vi "Fetch Measurement (Spectrum Emission Mask).vi"(0 "VISA resource name":refnum<visa-resource-name>, 5 "Timeout (10000 ms)":u32=10000, 11 "error in (no error)":errorcluster) -> (4 "VISA resource name out":refnum<visa-resource-name>, 6 "Measurement Data":dbl[](array[numeric]), 15 "error out":errorcluster)   [LabVIEW 2022 SP3, in "Agilent N934X Series.lvlib"]
doc: "Returns the results of last measurement (Spectrum Emission Mask) and does not initiate data acquisition.\n\nNote:\n\nUse this VI only with other low-level VIs. The high-level VIs automatically incorporate this functionality. This VI does not check the instrument status.\n\nThis VI is only applicable for N9321C, N9322C, N9323C, N9324C models."
uses:
  <instrlib>/Agilent N934X Series/Agilent N934X Series.lvlib
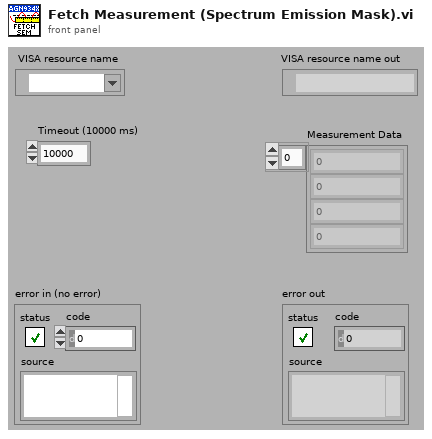
[diagram p1: front panel]
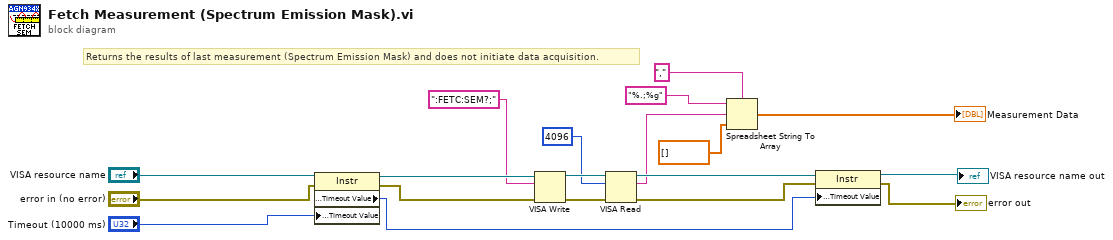
[diagram p0: block diagram]
diagram:
  # "Returns the results of last measurement (Spectrum Emission Mask) and does not initiate data acquisition."
  n1 = property on="Property Node" class="Instr"(reference="VISA resource name", error in="error in (no error)", "General Settings:Timeout Value"="Timeout (10000 ms)") -> (reference out=w17:refnum<visa-resource-name>, error out=w16:errorcluster, "General Settings:Timeout Value"=w18:u32)
  n2 = VISA Write(VISA resource name=w17, write buffer=":FETC:SEM?;", error in (no error)=w16) -> (VISA resource name out=w7:refnum<visa-resource-name>, error out=w8:errorcluster)  [unwired: 1 out]
  n3 = VISA Read(VISA resource name=w7, byte count=u32 4096, error in (no error)=w8) -> (VISA resource name out=w15:refnum<visa-resource-name>, read buffer=w5:string, error out=w12:errorcluster)  [unwired: 1 out]
  n4 = Spreadsheet String To Array(delimiter (Tab)=",", format string="%.;%g", spreadsheet string=w5, array type (2D Dbl)=dbl[] [] ("Measurement Data 2")) -> (array=→"Measurement Data":dbl[])
  n5 = property on="Property Node" class="Instr"(reference=w15, error in=w12, "General Settings:Timeout Value"=w18) -> (reference out=→"VISA resource name out":refnum<visa-resource-name>, error out=→"error out":errorcluster)
